vi "Agilent 3352X Series Frequency Sweep.vi"() -> ()   [LabVIEW 2019]
doc: "This example shows how to configure and enable a frequency sweep."
uses:
  <instrlib>/Agilent 3352X Series/Agilent 3352X Series.lvlib
panel:
  in  "Waveform Function (0: Sine)":i32(ring) items=["Sine"=0, "Square"=1, "Ramp"=2, "Noise"=3, "DC"=4, "Triangle"=5, "Pulse"=6, "Sinc"=11, "D-Lorentz"=12, "Gaussian"=13, "Expo Fall"=14, "Expo Rise"=15, "Haversine"=16]
  in  "Sweep Time (1 s)":dbl=1.0
  in  "Start Frequency (100 Hz)":dbl=100.0 format="%#.4f"
  in  "Stop  Frequency (1000 Hz)":dbl=1000.0 format="%#.4f"
  in  "Amplitude (0.1 Vpp)":dbl=0.1
  in  "VISA resource name":refnum<visa-resource-name>
  # "(c) 2011-2021 National Instruments.  ALL RIGHTS RESERVED."
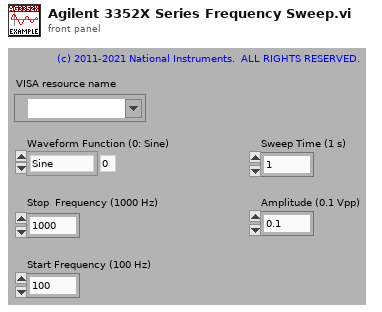
[diagram p1: front panel]
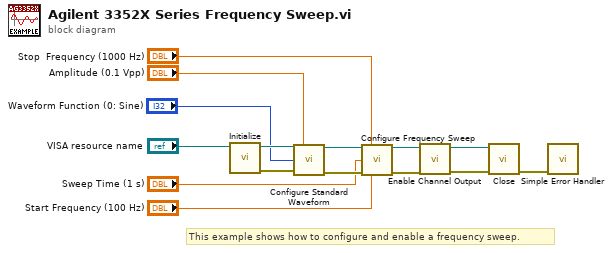
[diagram p0: block diagram]
diagram:
  # "This example shows how to configure and enable a frequency sweep."
  n1 = call <instrlib>:"Initialize.vi"("VISA resource name"="VISA resource name") -> ("error out"=w10:errorcluster, "VISA resource name out"=w11:refnum<visa-resource-name>)  [unwired: 4 in, 5 out]
  n2 = call <instrlib>:"Configure Standard Waveform.vi"("VISA resource name"=w11, "Amplitude (0.1 Vpp)"="Amplitude (0.1 Vpp)", "Waveform Function (0: Sine)"="Waveform Function (0: Sine)", "error in (no error)"=w10) -> ("VISA resource name out"=w9:refnum<visa-resource-name>, "error out"=w6:errorcluster)  [unwired: 6 in, 4 out]
  n3 = call <instrlib>:"Configure Frequency Sweep.vi"("VISA resource name"=w9, "Stop  Frequency (1000 Hz)"="Stop  Frequency (1000 Hz)", "Sweep Time (1 s)"="Sweep Time (1 s)", "error in (no error)"=w6, "Start Frequency (100 Hz)"="Start Frequency (100 Hz)") -> ("VISA resource name out"=w8:refnum<visa-resource-name>, "error out"=w7:errorcluster)  [unwired: 4 in, 5 out]
  n4 = call <instrlib>:"Enable Channel Output.vi"("error in (no error)"=w7, "VISA resource name"=w8) -> ("error out"=w13:errorcluster, "VISA resource name out"=w12:refnum<visa-resource-name>)  [unwired: 3 in, 5 out]
  n5 = call <instrlib>:"Close.vi"("error in (no error)"=w13, "VISA resource name"=w12) -> ("error out"=w15:errorcluster)  [unwired: 9 out]
  n6 = call <vilib>:"Simple Error Handler.vi"("error in (no error)"=w15) -> ()  [unwired: 1 in, 8 out]
